vi "PRL CALC Calculate Live Buffers in Access Buffer.vi"(9 "Sampling rate [Hz]":dbl, 10 "Access Buffer Size\n[hh:mm:ss]":dbl=18000.0 format="%<%H:%M:%S>t", 11 "Live Data Buffer Size\n[#data points]":i32=10) -> (1 "Actual Buffer Size":dbl=18000.0 format="%<%H:%M:%S>t", 2 "Buffer Mismatch":bool, 3 "Number of Live Buffers in Access Buffer":i32)   [LabVIEW 2013, in "PMU Recorder Light.lvlib"]
uses:
  PMU Recorder Light.lvlib
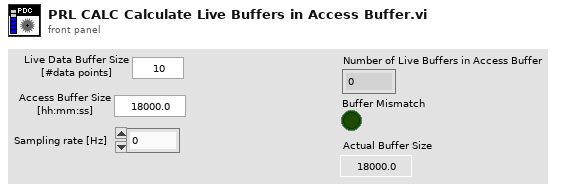
[diagram p1: front panel]
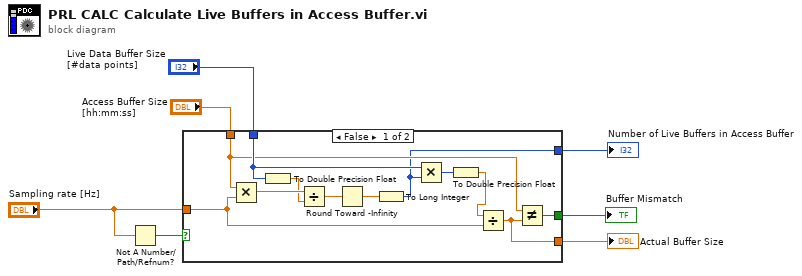
[diagram p0: block diagram]
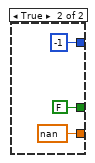
[diagram p2: hidden frame]
diagram:
  n1 = Not A Number/Path/Refnum?(number/path/refnum="Sampling rate [Hz]") -> (NaN/Path/Refnum?=w4:bool)
  n2 = case shown="False" w4 {
    tunnel: "Live Data Buffer Size\n[#data points]" -> [w13 _]
    tunnel: "Access Buffer Size\n[hh:mm:ss]" -> [w12 _]
    tunnel: "Sampling rate [Hz]" -> [w11 _]
    tunnel: [w10 FALSE] -> w2
    tunnel: [w9 -1] -> w3
    tunnel: [w8 nan] -> w1
    frame False {
      n3 = Multiply(x=w12, y=w11) -> (x*y=w19:dbl)
      n4 = To Double Precision Float(number=w13) -> (double precision float=w18:dbl)
      n5 = Divide(x=w19, y=w18) -> (x/y=w17:dbl)
      n6 = Round Toward -Infinity(1:w17) -> (0:w16:dbl)
      n7 = To Long Integer(number=w16) -> (32bit integer=w9:i32)
      n8 = Multiply(x=w13, y=w9) -> (x*y=w15:i32)
      n9 = To Double Precision Float(number=w15) -> (double precision float=w14:dbl)
      n10 = Divide(x=w14, y=w11) -> (x/y=w8:dbl)
      n11 = Not Equal?(x=w12, y=w8) -> (x != y?=w10:bool)
    }
    frame True {
    }
  }
  "Number of Live Buffers in Access Buffer" <- w3
  "Buffer Mismatch" <- w2
  "Actual Buffer Size" <- w1
